vi "Get Operating System Architecture.vi"(8 "error in (no error)":errorcluster, 11 "RT Management in":refnum<class "RT Management.lvclass">) -> (0 "error out":errorcluster, 2 "Operating System Architecture":string, 3 "RT Management out":refnum<class "RT Management.lvclass">)   [LabVIEW 2015, in "RT Management.lvlib" / "RT Management.lvclass"]
uses:
  RT Management.lvclass
  RT Management.lvclass/RT Management.ctl
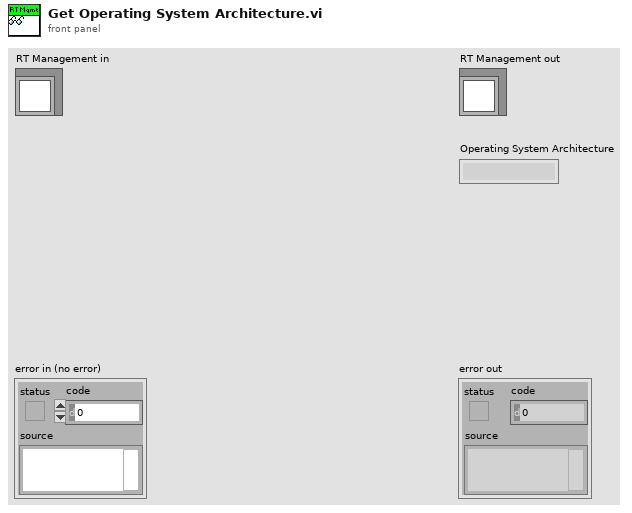
[diagram p1: front panel]
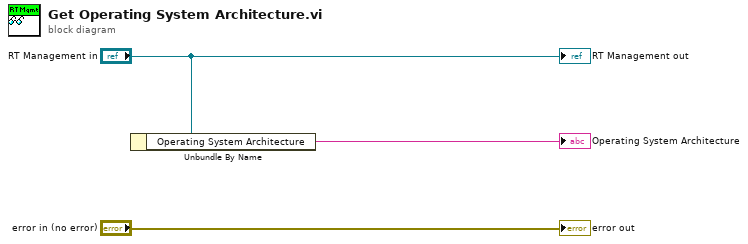
[diagram p0: block diagram]
diagram:
  n1 = Unbundle By Name("RT Management in") -> ("Operating System Architecture"=→"Operating System Architecture":string)
  "error out" <- "error in (no error)"
  "RT Management out" <- "RT Management in"
